vi "8_3.vi"() -> ()   [LabVIEW 2022 SP3]
panel:
  in  "OK Button":bool
  out "Waveform Chart":dbl(graph)
  in  "noise amplitude":dbl
  in  "dx":dbl
  in  "stop":bool
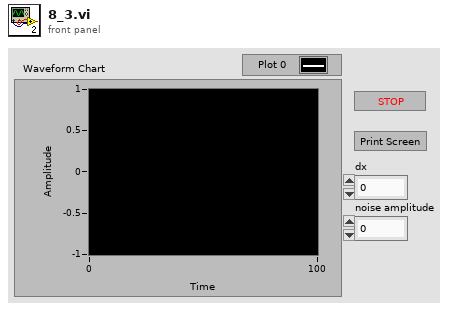
[diagram p1: front panel]
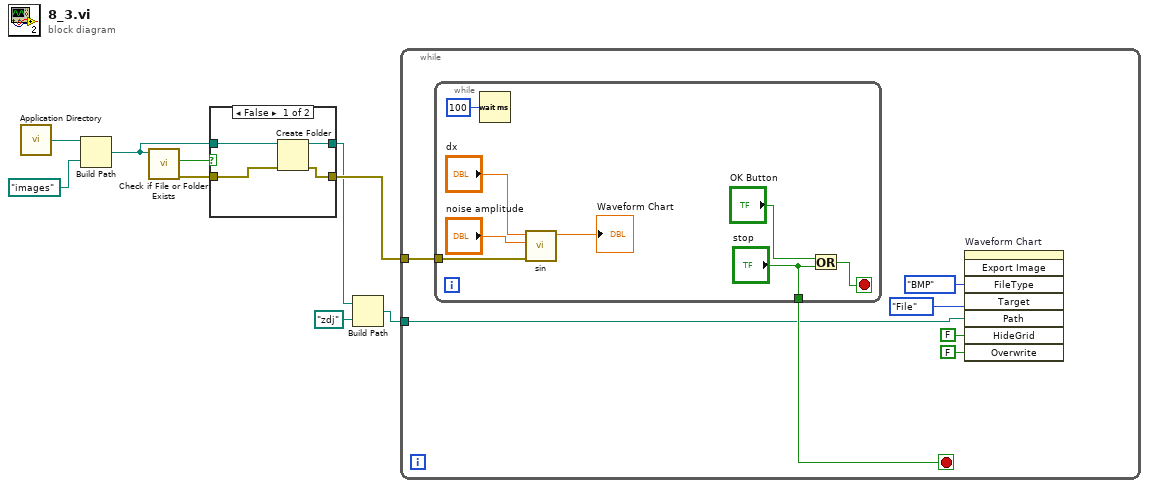
[diagram p0: block diagram]
diagram:
  n1 = call <vilib>:"Application Directory.vi"() -> ("Application Directory"=w9:path)
  n2 = Build Path(base path=w9, name or relative path=path "images") -> (appended path=w6:path)
  n3 = call <vilib>:"Check if File or Folder Exists.vi"("path"=w6) -> ("error out"=w5:errorcluster, "file or folder exists?"=w7:bool)  [unwired: 8 in, 1 out]
  n4 = case shown="False" w7 {
    tunnel: w6 -> [w13 w15]
    tunnel: w5 -> [w12 w14]
    tunnel: [w11 w15] -> w3
    tunnel: [w10 w14] -> w4
    frame False {
      n5 = Create Folder(path (use dialog)=w13, error in=w12) -> (created path=w11:path, error out=w10:errorcluster)  [unwired: 1 in, 1 out]
    }
    frame True {
    }
  }
  n6 = Build Path(base path=w3, name or relative path=path "zdj") -> (appended path=w1:path)
  n7 = while {
    tunnel: w4 -> [w22]
    tunnel: w1 -> [w16]
    stop <- w21 stop-if-true
    n8 = while {
      tunnel: w22 -> [w30]
      tunnel: ["stop"] -> w21
      stop <- w23 stop-if-true
      n9 = Wait (ms)(milliseconds to wait=u32 100) -> ()  [unwired: 1 out]
      n10 = call "sin.vi"("error constant"=w30, "noise amplitude"="noise amplitude", "dx"="dx") -> ("sin x"=→"Waveform Chart":dbl)  [unwired: 7 in, 1 out]
      n11 = Or(x="OK Button", y="stop") -> (x .or. y?=w23:bool)
    }
    n12 = invoke on="Waveform Chart" class="WFChart (strict)" method="Export Image"("FileType"=enum32{"BMP", "EPS", "EMF", "PICT"}."BMP" ("File Type"), "Target"=enum32{"File", "Clipboard"}."File", "Path"=w16, "HideGrid"=FALSE ("Hide Grid"), "Overwrite"=FALSE ("Always Overwrite")) -> ()  [unwired: 3 in, 8 out]
  }
